vi "AUTOFOCUS_read_QPD_signal_autofocus.vi"(6 "error in":errorcluster, 7 "i IR lost":i32, 8 "channel":bool, 9 "QPDcount":u32) -> (0 "error out":errorcluster, 2 "IR lost?":bool, 3 "i IR lost OUT":i32, 4 "QPDcount OUT":u32, 5 "QPD":dbl)   [LabVIEW 2015]
uses:
  GLOBAL/Global_FPGA.vi
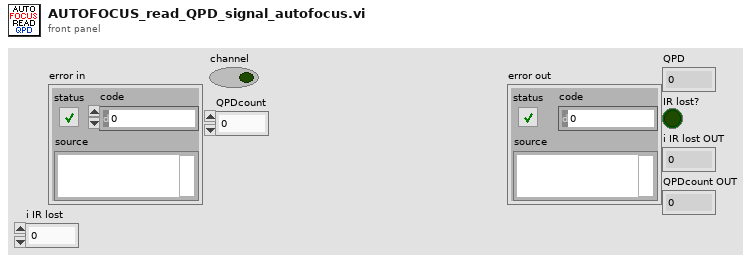
[diagram p1: front panel]
types:
  T1 = cluster{"X":sgl, "Y":sgl, "SUM":sgl, "count":u32}
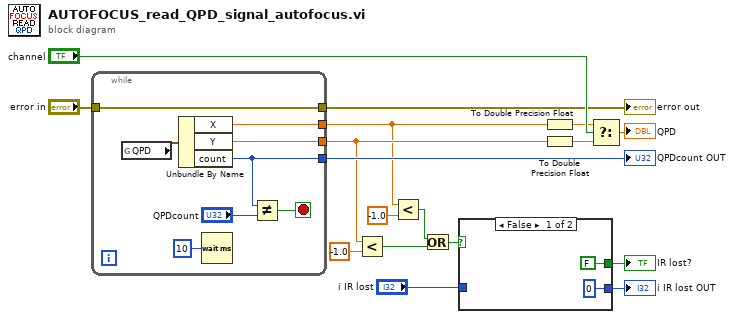
[diagram p0: block diagram]
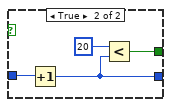
[diagram p2: hidden frame]
diagram:
  n1 = while {
    tunnel: [w24] -> w6
    tunnel: [w23] -> w4
    tunnel: [w21] -> w9
    tunnel: "error in" -> [w22]
    tunnel: [w22] -> w7
    stop <- w20 stop-if-true
    n2 = global read "Global_FPGA.vi" "QPD"() -> (w25:T1)
    n3 = Unbundle By Name(w25) -> ("X"=w23:sgl, "Y"=w24:sgl, "count"=w21:u32)
    n4 = Wait (ms)(milliseconds to wait=u32 10) -> ()  [unwired: 1 out]
    n5 = Not Equal?(x=w21, y="QPDcount") -> (x != y?=w20:bool)
  }
  "error out" <- w7
  "QPDcount OUT" <- w9
  n6 = Less?(x=w6, y=sgl -1.0) -> (x < y?=w2:bool)
  n7 = Less?(x=w4, y=sgl -1.0) -> (x < y?=w1:bool)
  n8 = Or(x=w1, y=w2) -> (x .or. y?=w3:bool)
  n9 = case shown="False" w3 {
    tunnel: "i IR lost" -> [_ w31]
    tunnel: [0 w30] -> w13
    tunnel: [FALSE w28] -> w12
    frame False {
    }
    frame True {
      n10 = Increment(x=w31) -> (x+1=w30:i32)
      n11 = Less?(x=20, y=w30) -> (x < y?=w28:bool)
    }
  }
  "IR lost?" <- w12
  "i IR lost OUT" <- w13
  n12 = To Double Precision Float(number=w4) -> (double precision float=w11:dbl)
  n13 = To Double Precision Float(number=w6) -> (double precision float=w10:dbl)
  n14 = Select(t=w11, s="channel", f=w10) -> (s? t:f=→"QPD":dbl)
